vi "Send.vi"(8 "error in (no error)":errorcluster, 9 "Caller Actor Name":string, 10 "Message Priority":T1, 11 "Message Transport":refnum<class "Message Transport Interface.lvclass">) -> (0 "error out":errorcluster)   [LabVIEW 2016, in "Stream Mediator.lvlib" / "Stop Msg.lvclass"]
doc: "--\nCopyright © 2017 Composed SystemsI All rights reserved.\n\nAuthor: Jon McBee <jon.mcbee@composed.io>\n\nThis library is provided \"AS IS\" ,WITHOUT WARRANTIES OR\nCONDITIONS OF ANY KIND, either express or implied.\n\nComposed Systems -- composed.io\n\nStream 0.0.1.1\nJon McBee - Composed Systems\nCopyright (c) 2017, Composed Systems"
uses:
  <userlib>/Composed Systems/Stream/Mediator/Classes/Message Command Stop/Stop Msg.lvclass
  <userlib>/Composed Systems/Stream/Mediator/Classes/Message Transport Interface/Message Priority.ctl
  <userlib>/Composed Systems/Stream/Mediator/Classes/Message Transport Interface/Message Transport Interface.lvclass
  C:/Program Files (x86)/National Instruments/LabVIEW 2016/user.lib/Composed Systems/Stream/Mediator/Classes/Message Command Interface/Command Message Interface.lvclass
  C:/Program Files (x86)/National Instruments/LabVIEW 2016/user.lib/Composed Systems/Stream/Mediator/Classes/Message Interface/Message Interface.lvclass
  <userlib>/Composed Systems/Stream/Mediator/Classes/Message Command Interface/Command Message Interface.lvclass/Command Message Interface.ctl
  <userlib>/Composed Systems/Stream/Mediator/Classes/Message Command Interface/Command Message Interface.lvclass
  <userlib>/Composed Systems/Stream/Mediator/Classes/Message Interface/Message Interface.lvclass
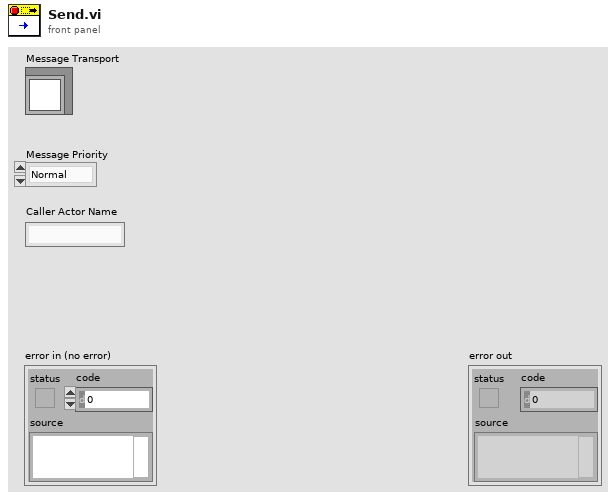
[diagram p1: front panel]
types:
  T1 = typedef "Stream Mediator.lvlib/Message Transport Interface.lvclass/Message Priority.ctl" = enum16{"Normal", "High"}
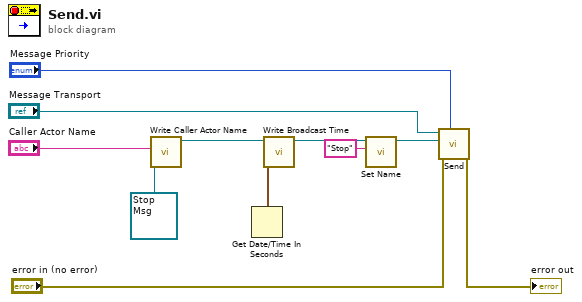
[diagram p0: block diagram]
diagram:
  n1 = call <userlib>:"Write Caller Actor Name.vi"("Caller Actor Name"="Caller Actor Name", "Command Message Interface in"=refnum<class "Stop Msg.lvclass"> refnum ("Stop Msg in")) -> ("Command Message Interface out"=w10:refnum<class "Stop Msg.lvclass">)  [unwired: 9 in]
  n2 = Get Date/Time In Seconds() -> (seconds since 1Jan1904=w6:timestamp)
  n3 = call <userlib>:"Write Broadcast Time.vi"("Broadcast Time"=w6, "Command Message Interface in"=w10) -> ("Command Message Interface out"=w5:refnum<class "Stop Msg.lvclass">)  [unwired: 9 in]
  n4 = call <userlib>:"Set Name.vi"("Name"="Stop", "Message Interface in"=w5) -> ("Message Interface out"=w4:refnum<class "Stop Msg.lvclass">)  [unwired: 8 in, 1 out]
  n5 = call-dynamic "Send.vi"("Message Priority"="Message Priority", "error in (no error)"="error in (no error)", "Message"=w4, "Message Transport Interface in"="Message Transport") -> ("error out"=→"error out":errorcluster)  [unwired: 5 in, 2 out]
